vi "De-Initialize.vi"(8 "error in (no error)":errorcluster, 11 "Device in":refnum<class "MB_TCP_Device.lvclass">) -> (0 "error out":errorcluster, 3 "Device out":refnum<class "MB_TCP_Device.lvclass">)   [LabVIEW 2023, in "MB_TCP_Device.lvclass"]
uses:
  MB_TCP_Device.lvclass
  MB_TCP_Device.lvclass/MB_TCP_Device.ctl
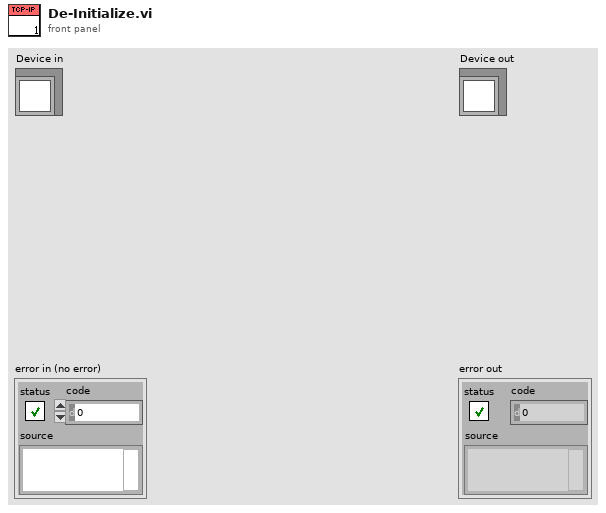
[diagram p1: front panel]
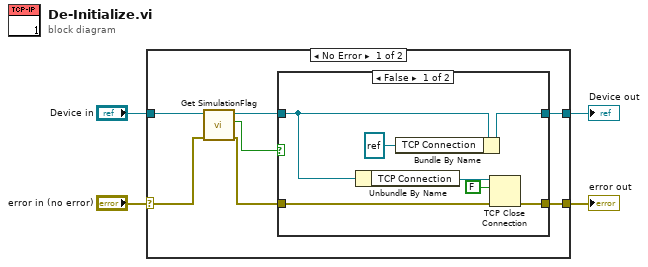
[diagram p0: block diagram]
diagram:
  n1 = case shown="No Error" "error in (no error)" {
    selector: "error in (no error)" -> [w7 w22]
    tunnel: [w11 w22] -> w3
    tunnel: [w10 w21] -> w1
    tunnel: "Device in" -> [w8 w21]
    frame No Error {
      n2 = call-dynamic "Get SimulationFlag.vi"("error in (no error)"=w7, "Device in"=w8) -> ("error out"=w6:errorcluster, "Simulation?"=w5:bool, "Device out"=w9:refnum<class "MB_TCP_Device.lvclass">)  [unwired: 7 in]
      n3 = case shown="False" w5 {
        tunnel: w9 -> [w18 w20]
        tunnel: w6 -> [w15 w19]
        tunnel: [w14 w19] -> w11
        tunnel: [w13 w20] -> w10
        frame False {
          n4 = Unbundle By Name(w18) -> ("TCP Connection"=w17:refnum<k5>)
          n5 = Bundle By Name(cluster=w18, "TCP Connection"=refnum<k5> refnum) -> (w13:refnum<class "MB_TCP_Device.lvclass">)
          n6 = TCP Close Connection(connection ID=w17, abort (F)=FALSE, error in (no error)=w15) -> (error out=w14:errorcluster)  [unwired: 1 out]
        }
        frame True {
        }
      }
    }
    frame Error {
    }
  }
  "error out" <- w3
  "Device out" <- w1
